vi "Finish.vi"   [LabVIEW 2016]
doc: "This VI is called just before exiting. It is expected to close I/O refnum, save collected data, etc."
uses:
  Robot Global Reference.vi
types:
  T1 = typedef "Joystick Reference.ctl" = cluster{"Driver Joystick":T2, "Operator Joystick":T2}
  T2 = typedef "WPI_JoystickDevRef.ctl" = cluster{"Device":T3}
  T3 = typedef "WPI_JoystickDeviceEnum.ctl" = enum16{"USB 0", "USB 1", "USB 2", "USB 3", "USB 4", "USB 5"}
  T4 = typedef "Drive Reference.ctl" = cluster{"RobotDriveDevRef":T5, "Drive PTO Solenoid":T10, "High Gear Solenoid":T10}
  T5 = typedef "WPI_RobotDriveDevRef.ctl" = cluster{"DevStatus":errorcluster, "Motors[]":T6[], "Square Inputs":bool, "Max Output":dbl}
  T6 = typedef "WPI_MotorControlDeviceRef.ctl" = cluster{"DeviceStatus":errorcluster, "Type":T7, "PWM":cluster{"PWM Channel":T8, "DeadBand":T9}, "CAN":cluster{"Device Number":u8, "SetOutput VI Ref":variant, "GetOutput VI Ref":variant, "Enable VI Ref":variant, "Disable VI Ref":variant, "Data":variant}, "Invert":bool}
  T7 = typedef "WPI_MotorControlType.ctl" = enum16{"PWM", "CAN"}
  T8 = typedef "FPGA_DIOPWMChannel.ctl" = enum8{"PWM 0", "PWM 1", "PWM 2", "PWM 3", "PWM 4", "PWM 5", "PWM 6", "PWM 7", "PWM 8", "PWM 9", "PWM MXP 0", "PWM MXP 1", "PWM MXP 2", "PWM MXP 3", "PWM MXP 4", "PWM MXP 5", "PWM MXP 6", "PWM MXP 7", "PWM MXP 8", "PWM MXP 9", "Invalid"}
  T9 = typedef "WPI_PWMDeadband.ctl" = cluster{"Name":string, "maxPositivePwm":i32, "minPositivePwm":i32, "centerPwm":i32, "maxNegativePwm":i32, "minNegativePwm":i32, "angularRange":u16}
  T10 = typedef "WPI_SolenoidDevRef.ctl" = cluster{"DevStatus":errorcluster, "Pneumatics Control Module":u8, "Forward Solenoid Channel":T11, "Reverse Solenoid Channel":T11}
  T11 = typedef "WPI_SolenoidChannel.ctl" = enum8{"Solenoid 0", "Solenoid 1", "Solenoid 2", "Solenoid 3", "Solenoid 4", "Solenoid 5", "Solenoid 6", "Solenoid 7", "Invalid"}
  T12 = typedef "Sensor Reference.ctl" = cluster{"LeftMotorEncoderRef":T13, "RightMotorEncoderRef":T13, "I2C Gyro":T17, "Left Shooter Wheel Encoder":T13, "Ultrasonic AIDeviceRef":T19}
  T13 = typedef "WPI_EncoderDevRef.ctl" = cluster{"DevStatus":errorcluster, "EncoderIndex":T14, "CounterIndex":T15, "DistancePerCount":dbl, "Decoding Type":T16}
  T14 = typedef "FPGA_EncoderIdx.ctl" = enum8{"Enc 0", "Enc 1", "Enc 2", "Enc 3", "Enc 4", "Enc 5", "Enc 6", "Enc 7", "Invalid"}
  T15 = typedef "FPGA_CounterCtrSystemIndex.ctl" = enum8{"Ctr 0", "Ctr 1", "Ctr 2", "Ctr 3", "Ctr 4", "Ctr 5", "Ctr 6", "Ctr 7", "Invalid"}
  T16 = typedef "WPI_EncoderType.ctl" = enum16{"1x", "2x", "4x"}
  T17 = typedef "WPI_I2CDevRef.ctl" = cluster{"DevStatus":errorcluster, "Device Address":u8, "Handle":i32, "I2C Bus":T18}
  T18 = typedef "i2c_bus.ctl" = enum16{"I2C On-Board", "I2C MXP", "Invalid"}
  T19 = typedef "WPI_AnalogChannelDevRef.ctl" = cluster{"DevStatus":errorcluster, "Analog Channel":T20}
  T20 = typedef "FPGA_AIChannel.ctl" = enum8{"AI 0", "AI 1", "AI 2", "AI 3", "AI MXP 0", "AI MXP 1", "AI MXP 2", "AI MXP 3", "Invalid"}
  T21 = typedef "Shoot Reference.ctl" = cluster{"Shooter Wheel Left":T6, "Shooter Wheel Right":T6, "Acquisition Conveyor Motor DevRef":T6, "Hopper Beater Bar Motor DevRef":T6}
  T22 = typedef "Gear Reference.ctl" = cluster{"Gear Ejection Cylinder":T10, "Door Ejection Cylinder":T10}
  T23 = typedef "Light Reference.ctl" = cluster{"SerialPortRef":T24}
  T24 = typedef "WPI_SerialPortRef.ctl" = cluster{"DevStatus":errorcluster, "Serial Port Name":refnum<visa-resource-name>}
  T25 = cluster{"Joystick Reference":T1, "Drive Reference":T4, "Sensor Reference":T12, "Shoot + Aquisition Reference":T21, "Gear Reference":T22, "Acquisition Conveyor Motor DevRef":T6, "Lights":T23}
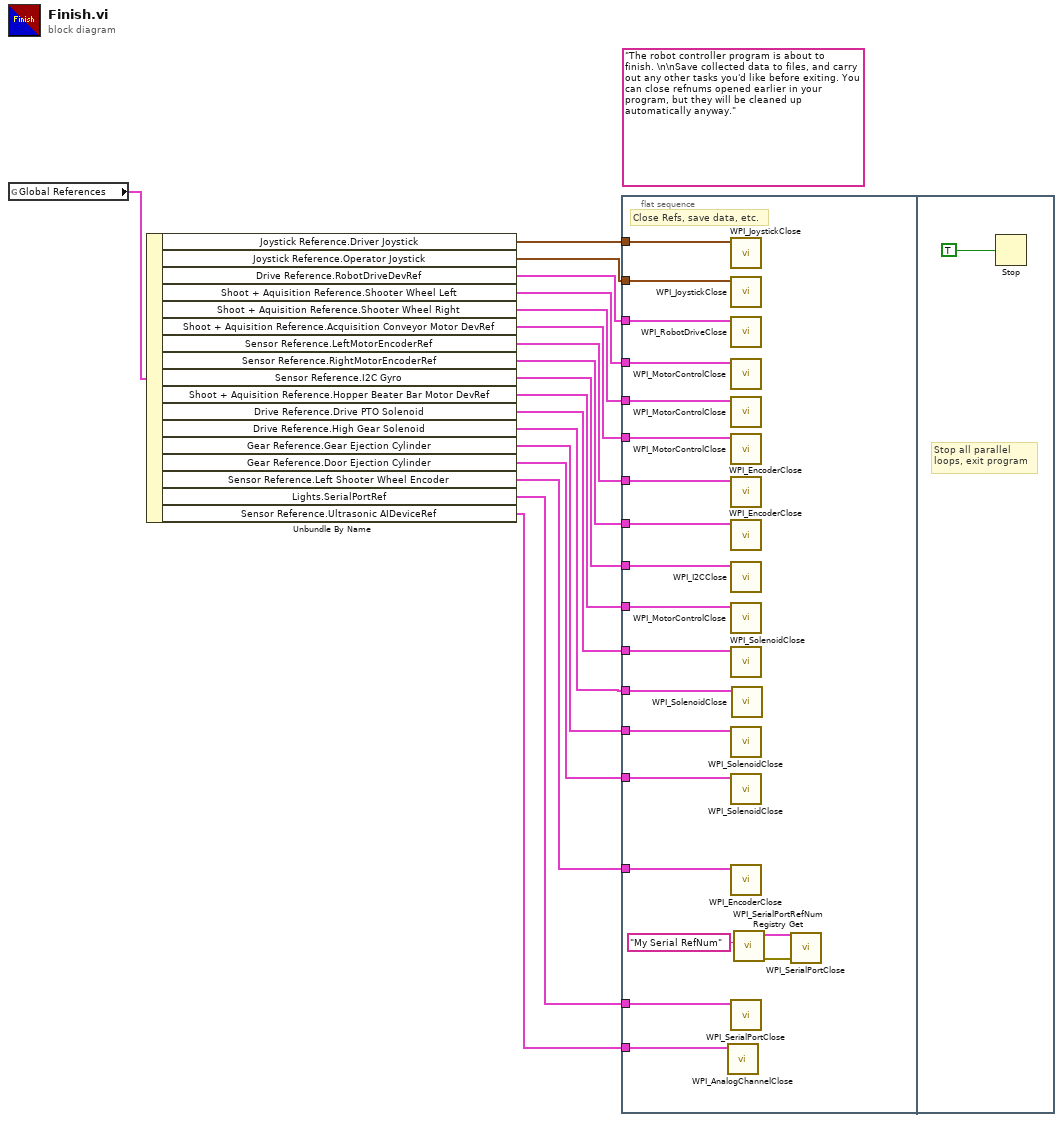
[diagram p0: block diagram]
diagram:
  (unwired) "The robot controller program is about to finish. \n\nSave collected data to files, and carry out any other tasks you'd like before exiting. You can close refnums opened earlier in your program, but they will be cleaned up automatically anyway."
  n1 = global read "Robot Global Reference.vi" "Global References"() -> (w18:T25)
  n2 = Unbundle By Name(w18) -> ("Joystick Reference.Driver Joystick"=w17:T2, "Joystick Reference.Operator Joystick"=w16:T2, "Drive Reference.RobotDriveDevRef"=w15:T5, "Shoot + Aquisition Reference.Shooter Wheel Left"=w14:T6, "Shoot + Aquisition Reference.Shooter Wheel Right"=w12:T6, "Shoot + Aquisition Reference.Acquisition Conveyor Motor DevRef"=w13:T6, "Sensor Reference.LeftMotorEncoderRef"=w11:T13, "Sensor Reference.RightMotorEncoderRef"=w10:T13, "Sensor Reference.I2C Gyro"=w9:T17, "Shoot + Aquisition Reference.Hopper Beater Bar Motor DevRef"=w8:T6, "Drive Reference.Drive PTO Solenoid"=w7:T10, "Drive Reference.High Gear Solenoid"=w3:T10, "Gear Reference.Gear Ejection Cylinder"=w6:T10, "Gear Reference.Door Ejection Cylinder"=w5:T10, "Sensor Reference.Left Shooter Wheel Encoder"=w4:T13, "Lights.SerialPortRef"=w2:T24, "Sensor Reference.Ultrasonic AIDeviceRef"=w1:T19)
  n3 = flat-sequence {
    tunnel: w17 -> [w38]
    tunnel: w16 -> [w37]
    tunnel: w15 -> [w36]
    tunnel: w14 -> [w35]
    tunnel: w13 -> [w34]
    tunnel: w12 -> [w33]
    tunnel: w11 -> [w32]
    tunnel: w10 -> [w31]
    tunnel: w9 -> [w30]
    tunnel: w8 -> [w29]
    tunnel: w7 -> [w28]
    tunnel: w6 -> [w27]
    tunnel: w5 -> [w26]
    tunnel: w4 -> [w25]
    tunnel: w3 -> [w24]
    tunnel: w2 -> [w23]
    tunnel: w1 -> [w19]
    frame #0 {
      # "Close Refs, save data, etc."
      n4 = call <vilib>:"WPI_AnalogChannelClose.vi"("AIDeviceRef"=w19) -> ()  [unwired: 10 in, 1 out]
      n5 = call <vilib>:"WPI_JoystickClose.vi"("JoystickDevRef"=w38) -> ()  [unwired: 11 out]
      n6 = call <vilib>:"WPI_JoystickClose.vi"("JoystickDevRef"=w37) -> ()  [unwired: 11 out]
      n7 = call <vilib>:"WPI_RobotDriveClose.vi"("RobotDriveDevRef"=w36) -> ()  [unwired: 1 in, 10 out]
      n8 = call <vilib>:"WPI_MotorControlClose.vi"("MotorControlDevRef"=w35) -> ()  [unwired: 10 in, 1 out]
      n9 = call <vilib>:"WPI_MotorControlClose.vi"("MotorControlDevRef"=w33) -> ()  [unwired: 10 in, 1 out]
      n10 = call <vilib>:"WPI_MotorControlClose.vi"("MotorControlDevRef"=w34) -> ()  [unwired: 10 in, 1 out]
      n11 = call <vilib>:"WPI_EncoderClose.vi"("EncoderDevRef"=w32) -> ()  [unwired: 10 in, 1 out]
      n12 = call <vilib>:"WPI_EncoderClose.vi"("EncoderDevRef"=w31) -> ()  [unwired: 10 in, 1 out]
      n13 = call <vilib>:"WPI_I2CClose.vi"("I2CDevRef"=w30) -> ()  [unwired: 10 in, 1 out]
      n14 = call <vilib>:"WPI_MotorControlClose.vi"("MotorControlDevRef"=w29) -> ()  [unwired: 10 in, 1 out]
      n15 = call <vilib>:"WPI_SolenoidClose.vi"("SolenoidDevRef"=w28) -> ()  [unwired: 10 in, 1 out]
      n16 = call <vilib>:"WPI_SolenoidClose.vi"("SolenoidDevRef"=w27) -> ()  [unwired: 10 in, 1 out]
      n17 = call <vilib>:"WPI_SolenoidClose.vi"("SolenoidDevRef"=w26) -> ()  [unwired: 10 in, 1 out]
      n18 = call <vilib>:"WPI_EncoderClose.vi"("EncoderDevRef"=w25) -> ()  [unwired: 10 in, 1 out]
      n19 = call <vilib>:"WPI_SerialPortClose.vi"("SerialPortRef"=w23) -> ()  [unwired: 10 in, 1 out]
      n20 = call <vilib>:"WPI_SolenoidClose.vi"("SolenoidDevRef"=w24) -> ()  [unwired: 10 in, 1 out]
      n21 = call <vilib>:"WPI_SerialPortRefNum Registry Get.vi"("refnum name"="My Serial RefNum") -> ("error out"=w21:errorcluster, "SerialPortRef"=w20:T24)  [unwired: 9 in]
      n22 = call <vilib>:"WPI_SerialPortClose.vi"("error in (no error)"=w21, "SerialPortRef"=w20) -> ()  [unwired: 9 in, 1 out]
    }
    frame #1 {
      # "Stop all parallel\nloops, exit program"
      n23 = Stop(stop? (T)=TRUE ("Quit")) -> ()
    }
  }
